vi "CVT Load Tag List.vi"(8 "error in":errorcluster, 10 "Target Name":string, 11 "TCE Config File Path":path) -> (0 "error out":errorcluster, 3 "CVT Tag List":T1[](array[typedef]))   [LabVIEW 2020, in "Current Value Table(Rebuild).lvlib"]
uses:
  _SubVIs/TypeDefs/cvt_Tag Configuration.ctl
  _SubVIs/TypeDefs/cvt_Data Types.ctl
  Current Value Table(Rebuild).lvlib
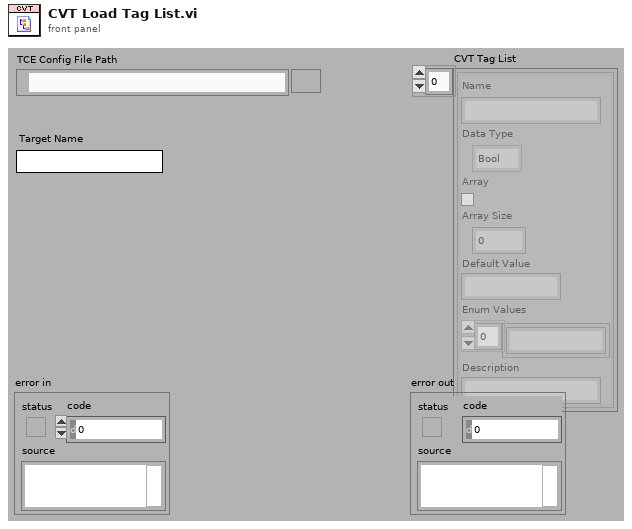
[diagram p1: front panel]
types:
  T1 = typedef "Current Value Table(Rebuild).lvlib/cvt_Tag Configuration.ctl" = cluster{"Name":string, "Data Type":T2, "Array":bool, "Size":u32, "Default":string, "Enum":string[], "Description":string}
  T2 = typedef "Current Value Table(Rebuild).lvlib/cvt_Data Types.ctl" = enum16{"Bool", "U8", "I32", "Double", "String", "Enum"}
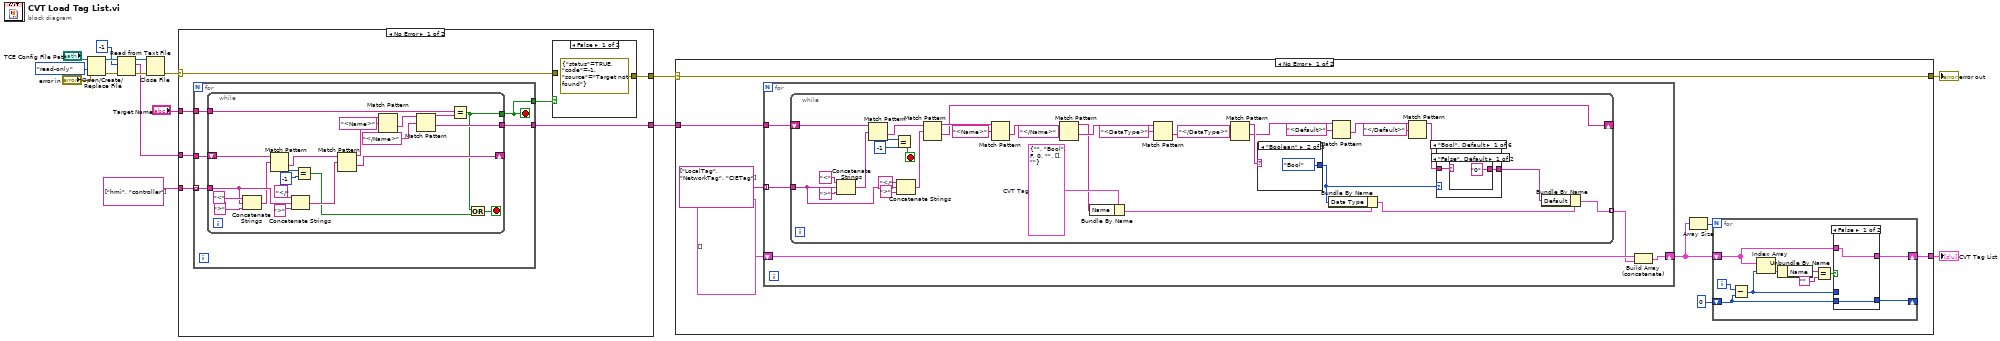
[diagram p0: block diagram]
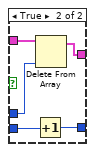
[diagram p2: hidden frame]
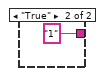
[diagram p3: hidden frame]
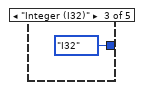
[diagram p10: hidden frame]
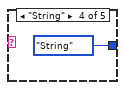
[diagram p11: hidden frame]
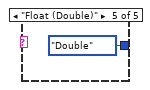
[diagram p12: hidden frame]
diagram:
  n1 = Open/Create/Replace File(file path (use dialog)="TCE Config File Path", error in="error in", access (0:read/write)=enum16{"read/write", "read-only", "write-only"}."read-only") -> (refnum out=w14:refnum<file>, error out=w13:errorcluster)  [unwired: 4 out]
  n2 = Read from Text File(file (use dialog)=w14, count=-1, error in=w13) -> (refnum out=w11:refnum<file>, text=w8:string, error out=w10:errorcluster)  [unwired: 2 out]
  n3 = Close File(refnum=w11, error in=w10) -> (error out=w9:errorcluster)  [unwired: 1 out]
  n4 = case shown="No Error" w9 {
    selector: w9 -> [w19 w53]
    tunnel: w8 -> [w23 _]
    tunnel: string[] ["hmi", "controller"] -> [w22 _]
    tunnel: "Target Name" -> [w21 _]
    tunnel: [w18 w53] -> w4
    tunnel: [w17 _] -> w5
    frame No Error {
      n5 = for {
        tunnel: w23 -> [w30]
        tunnel: w22 -> [w29] mode=indexing
        tunnel: w21 -> [w28]
        tunnel: [w27] -> w17
        tunnel: [w26] -> w20
        stop <- w26 stop-if-true
        n6 = while {
          tunnel: w29 -> [w49]
          shift-right: [w39] -> _
          shift-left: w30 -> [w52]
          tunnel: w28 -> [w33]
          tunnel: [w32] -> w27
          tunnel: [w31] -> w26
          stop <- w41 stop-if-true
          n7 = Concatenate Strings("<", w49, ">") -> (w46:string)
          n8 = Match Pattern(string=w52, regular expression=w46) -> (after substring=w43:string, offset past match=w45:i32)  [unwired: 3 out]
          n9 = Concatenate Strings("</" ("string"), w49, ">" ("string")) -> (w42:string)
          n10 = Equal?(x=w45, y=-1 ("offset past match")) -> (x = y?=w40:bool)
          n11 = Match Pattern(string=w43, regular expression=w42) -> (before substring=w37:string, after substring=w39:string)  [unwired: 3 out]
          n12 = Match Pattern(string=w37, regular expression="<Name>") -> (after substring=w36:string)  [unwired: 4 out]
          n13 = Match Pattern(string=w36, regular expression="</Name>") -> (before substring=w34:string, after substring=w32:string)  [unwired: 3 out]
          n14 = Equal?(x=w33, y=w34) -> (x = y?=w31:bool)
          n15 = Or(x=w31, y=w40) -> (x .or. y?=w41:bool)
        }
      }
      n16 = case shown="False" w20 {
        tunnel: w19 -> [_ w25]
        tunnel: [errorcluster {"status"=TRUE, "code"=-1, "source"="Target not found"} ("error IO") w25] -> w18
        frame False {
        }
        frame True {
        }
      }
    }
    frame Error {
    }
  }
  n17 = case shown="No Error" w4 {
    selector: w4 -> [w54 w131]
    tunnel: w5 -> [w60 _]
    tunnel: [w56 _] -> w3
    tunnel: [w54 w131] -> w1
    frame No Error {
      n18 = for {
        tunnel: string[] ["LocalTag", "NetworkTag", "CIETag"] -> [w82] mode=indexing
        tunnel: w60 -> [w83]
        shift-right: [w79] -> w55
        shift-left: T1[] [] ("Tag List") -> [w81]
        n19 = while {
          tunnel: w82 -> [w105]
          shift-right: [w84] -> _
          shift-left: w83 -> [w117]
          tunnel: [w104] -> w80 mode=indexing
          stop <- w107 stop-if-true
          w100 = T1 {"Name"="", "Data Type"=enum."Bool", "Array"=FALSE, "Size"=0, "Default"="", "Enum"=[], "Description"=""}  # CVT Tag
          n20 = Concatenate Strings("<" ("string"), w105, ">" ("string")) -> (w114:string)
          n21 = Match Pattern(string=w117, regular expression=w114) -> (after substring=w113:string, offset past match=w109:i32)  [unwired: 3 out]
          n22 = Equal?(x=w109, y=-1) -> (x = y?=w107:bool)
          n23 = Concatenate Strings("</" ("string"), w105, ">" ("string")) -> (w110:string)
          n24 = Match Pattern(string=w113, regular expression=w110) -> (before substring=w106:string, after substring=w84:string)  [unwired: 3 out]
          n25 = Match Pattern(string=w106, regular expression="<Name>") -> (after substring=w103:string)  [unwired: 4 out]
          n26 = Match Pattern(string=w103, regular expression="</Name>") -> (before substring=w88:string, after substring=w96:string)  [unwired: 3 out]
          n27 = Bundle By Name(cluster=w100, "Name"=w88) -> (w94:T1)
          n28 = Match Pattern(string=w96, regular expression="<DataType>") -> (after substring=w97:string)  [unwired: 4 out]
          n29 = Match Pattern(string=w97, regular expression="</DataType>") -> (before substring=w95:string, after substring=w90:string)  [unwired: 3 out]
          n30 = case shown="\"Boolean\"" w95 {
            tunnel: [_ cvt_Data_Types."Bool" ("Data Type") cvt_Data_Types."I32" ("Data Type") cvt_Data_Types."String" ("Data Type") cvt_Data_Types."Double" ("Data Type")] -> w87
            frame Default {
            }
            frame "Boolean" {
            }
            frame "Integer (I32)" {
            }
            frame "String" {
            }
            frame "Float (Double)" {
            }
          }
          n31 = Bundle By Name(cluster=w94, "Data Type"=w87) -> (w85:T1)
          n32 = Match Pattern(string=w90, regular expression="<Default>") -> (after substring=w93:string)  [unwired: 4 out]
          n33 = Match Pattern(string=w93, regular expression="</Default>") -> (before substring=w89:string)  [unwired: 4 out]
          n34 = case shown="\"Bool\", Default" w87 {
            tunnel: w89 -> [w119 w122 w123 w124 w125 w126]
            tunnel: [w118 w122 w123 w124 w125 w126] -> w86
            frame "Bool", Default {
              n35 = case shown="\"False\", Default" w119 {
                tunnel: ["0" "1"] -> w118
                frame "False", Default {
                }
                frame "True" {
                }
              }
            }
            frame "U8" {
            }
            frame "I32" {
            }
            frame "Double" {
            }
            frame "String" {
            }
            frame "Enum" {
            }
          }
          n36 = Bundle By Name(cluster=w85, "Default"=w86) -> (w104:T1)
        }
        n37 = Build Array (concatenate)(w81, w80) -> (w79:T1[])
      }
      n38 = Array Size(array=w55) -> (size(s)=w57:i32)
      n39 = for {
        N: w57 -> [_]
        shift-right: [w64] -> w56
        shift-left: w55 -> [w66]
        shift-right: [w62] -> _
        shift-left: 0 -> [w63]
        i -> [w71]
        n40 = Subtract(x=w71, y=w63) -> (x-y=w65:i32)
        n41 = Index Array(array=w66, index=w65) -> (element=w70:T1)
        n42 = Unbundle By Name(w70) -> ("Name"=w69:string)
        n43 = Equal?(x=w69, y="") -> (x = y?=w67:bool)
        n44 = case shown="False" w67 {
          tunnel: w66 -> [w72 w78]
          tunnel: w65 -> [_ w77]
          tunnel: [w72 w76] -> w64
          tunnel: w63 -> [w73 w75]
          tunnel: [w73 w74] -> w62
          frame False {
          }
          frame True {
            n45 = Increment(x=w75) -> (x+1=w74:i32)
            n46 = Delete From Array(array=w78, index=w77) -> (array with subset deleted=w76:T1[])  [unwired: 1 in, 1 out]
          }
        }
      }
    }
    frame Error {
    }
  }
  "CVT Tag List" <- w3
  "error out" <- w1
